vi "sub vi - defrag tdms v1.vi"(11 "panel id":string) -> (0 "error out":errorcluster)   [LabVIEW 2017]
uses:
  Global 1.vi
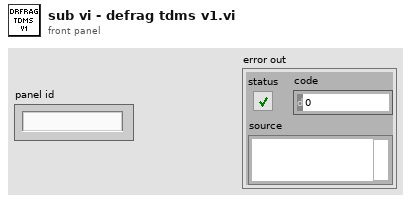
[diagram p1: front panel]
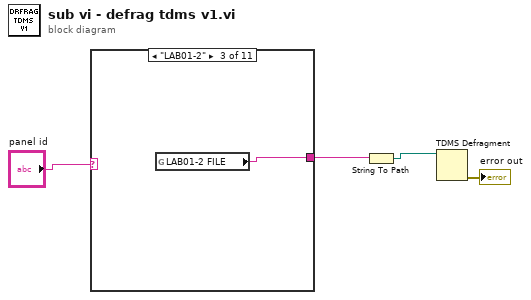
[diagram p0: block diagram]
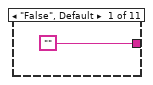
[diagram p2: hidden frame]
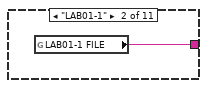
[diagram p3: hidden frame]
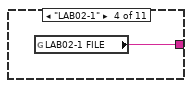
[diagram p4: hidden frame]
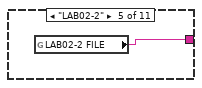
[diagram p5: hidden frame]
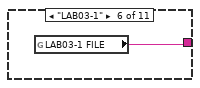
[diagram p6: hidden frame]
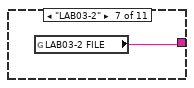
[diagram p7: hidden frame]
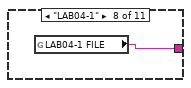
[diagram p8: hidden frame]
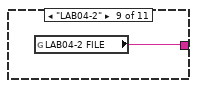
[diagram p9: hidden frame]
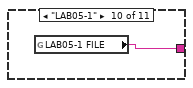
[diagram p10: hidden frame]
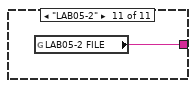
[diagram p11: hidden frame]
diagram:
  n1 = case shown="\"LAB01-2\"" "panel id" {
    tunnel: ["" w6 w7 w8 w9 w10 w11 w12 w13 w14 w15] -> w3
    frame "False", Default {
    }
    frame "LAB01-1" {
      n2 = global read "Global 1.vi" "LAB01-1 FILE"() -> (w6:string)
    }
    frame "LAB01-2" {
      n3 = global read "Global 1.vi" "LAB01-2 FILE"() -> (w7:string)
    }
    frame "LAB02-1" {
      n4 = global read "Global 1.vi" "LAB02-1 FILE"() -> (w8:string)
    }
    frame "LAB02-2" {
      n5 = global read "Global 1.vi" "LAB02-2 FILE"() -> (w9:string)
    }
    frame "LAB03-1" {
      n6 = global read "Global 1.vi" "LAB03-1 FILE"() -> (w10:string)
    }
    frame "LAB03-2" {
      n7 = global read "Global 1.vi" "LAB03-2 FILE"() -> (w11:string)
    }
    frame "LAB04-1" {
      n8 = global read "Global 1.vi" "LAB04-1 FILE"() -> (w12:string)
    }
    frame "LAB04-2" {
      n9 = global read "Global 1.vi" "LAB04-2 FILE"() -> (w13:string)
    }
    frame "LAB05-1" {
      n10 = global read "Global 1.vi" "LAB05-1 FILE"() -> (w14:string)
    }
    frame "LAB05-2" {
      n11 = global read "Global 1.vi" "LAB05-2 FILE"() -> (w15:string)
    }
  }
  n12 = String To Path(string=w3) -> (path=w2:path)
  n13 = TDMS Defragment(7:w2) -> (0:→"error out":errorcluster)  [unwired: 1 in]
